vi "Create Combination.vi"(9 "Array":dbl[](array[numeric]), 10 "Index":i32, 11 "Temp Combination":dbl[](array[numeric])) -> (5 "Combinations Out":dbl[][](array[numeric]))   [LabVIEW 2018]
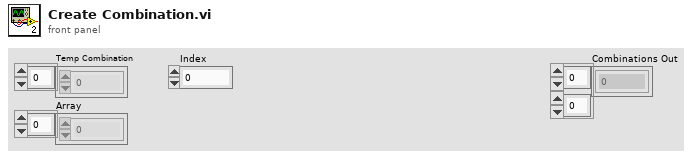
[diagram p1: front panel]
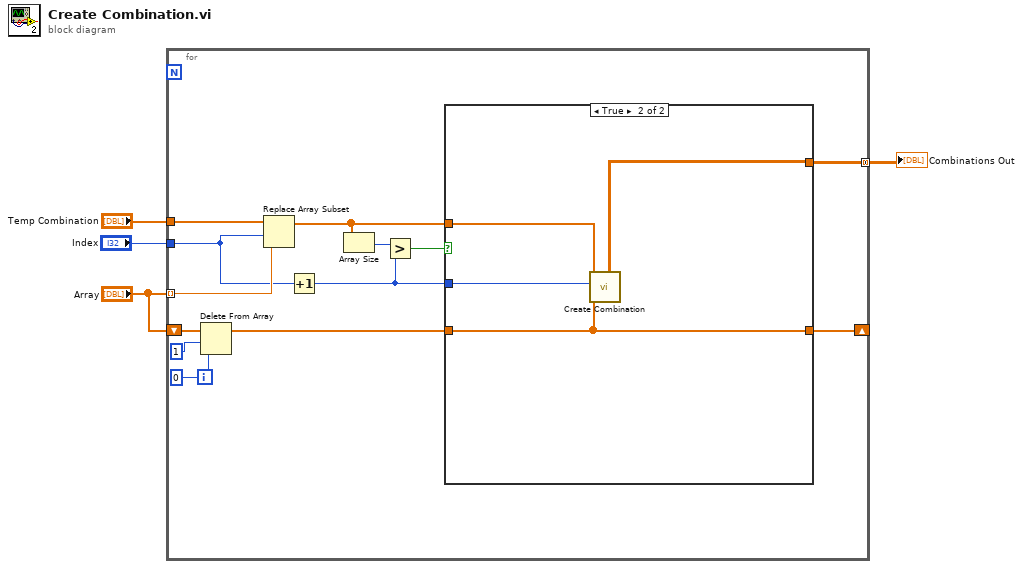
[diagram p0: block diagram]
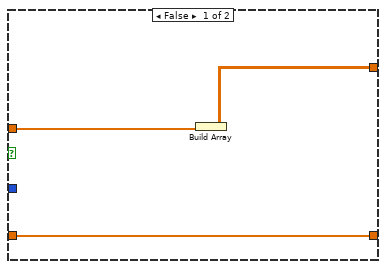
[diagram p2: hidden frame]
diagram:
  n1 = for {
    tunnel: "Temp Combination" -> [w16]
    tunnel: "Array" -> [w15] mode=indexing
    shift-right: [w7] -> _
    shift-left: "Array" -> [w17]
    tunnel: "Index" -> [w11]
    tunnel: [w5] -> w1 mode=concatenating
    n2 = Delete From Array(array=w17, length=1, index=0) -> (array with subset deleted=w8:dbl[])  [unwired: 1 out]
    n3 = Replace Array Subset(array=w16, new element=w15, index=w11) -> (w9:dbl[])
    n4 = Increment(x=w11) -> (x+1=w6:i32)
    n5 = Array Size(array=w9) -> (size(s)=w12:i32)
    n6 = Greater?(x=w12, y=w6) -> (0:w10:bool)
    n7 = case shown="True" w10 {
      tunnel: w9 -> [w19 w23]
      tunnel: w8 -> [w20 w24]
      tunnel: [w20 w24] -> w7
      tunnel: [w18 w22] -> w5
      tunnel: w6 -> [_ w21]
      frame False {
        n8 = Build Array(w19) -> (w18:dbl[][])
      }
      frame True {
        n9 = call "Create Combination.vi"("Array"=w24, "Index"=w21, "Temp Combination"=w23) -> ("Combinations Out"=w22:dbl[][])  [unwired: 8 in]
      }
    }
  }
  "Combinations Out" <- w1
